vi "Shooter Mode Selector.vi"(9 "Manual":bool, 10 "Auto":bool) -> (2 "Mode":T1)   [LabVIEW 2016]
uses:
  Common Code/Shooter Modes.ctl
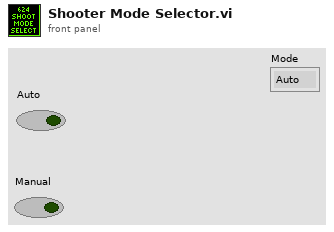
[diagram p1: front panel]
types:
  T1 = typedef "Shooter Modes.ctl" = enum16{"Auto", "Manual"}
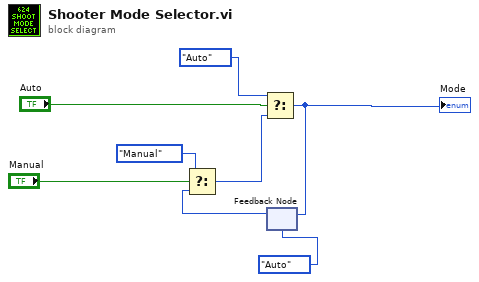
[diagram p0: block diagram]
diagram:
  n1 = feedback #1(Shooter_Modes."Auto" ("Shooter Modes")) -> (w2:T1)
  n2 = Select(t=Shooter_Modes."Manual" ("Shooter Modes"), s="Manual", f=w2) -> (s? t:f=w5:T1)
  n3 = Select(t=Shooter_Modes."Auto" ("Shooter Modes"), s="Auto", f=w5) -> (s? t:f=w3:T1)
  "Mode" <- w3
  n4 = feedback-in #1(w3) -> ()
